vi "Example CaseStructure 2.vi"(8 "Error In":errorcluster) -> (0 "Error Out":errorcluster, 1 "signal out":waveform(dbl), 3 "appended array":waveform(dbl)[](array[waveform]))   [LabVIEW 2014]
uses:
  <vilib>/measure/NI_MABase.lvlib
panel:
  out "Boolean 3":bool
  out "Boolean 2":bool
  in  "Boolean":bool
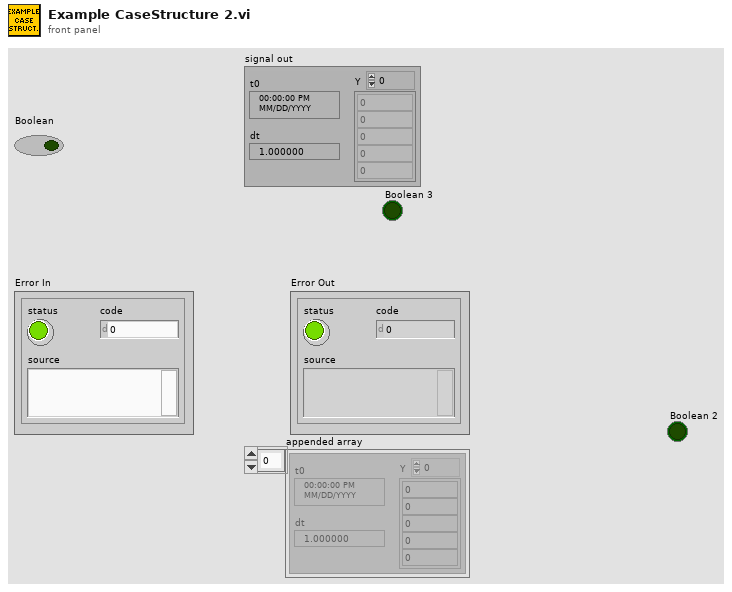
[diagram p1: front panel]
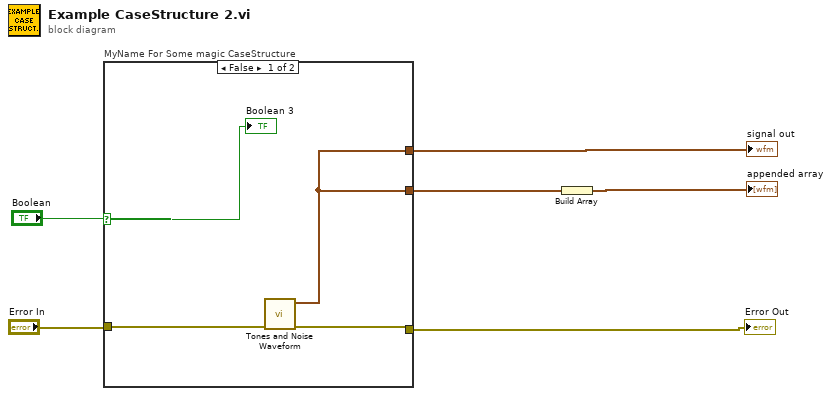
[diagram p0: block diagram]
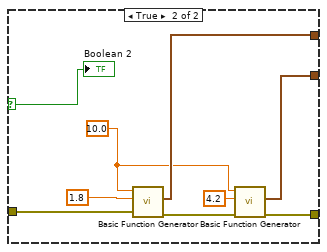
[diagram p2: hidden frame]
diagram:
  n1 = case "MyName For Some magic CaseStructure" shown="False" "Boolean" {
    selector: "Boolean" -> [w7 w11]
    tunnel: "Error In" -> [w10 w19]
    tunnel: [w9 w17] -> w1
    tunnel: [w8 w14] -> w4
    tunnel: [w8 w13] -> w3
    frame False {
      n2 = call <vilib>:"Tones and Noise Waveform.vi"("error in (no error)"=w10) -> ("error out"=w9:errorcluster, "signal out"=w8:waveform(dbl))  [unwired: 9 in]
      "Boolean 3" <- w7
    }
    frame True {
      w12 = 10.0 ("frequency")
      n3 = call <vilib>:"Basic Function Generator.vi"("error in (no error)"=w19, "amplitude"=1.8, "frequency"=w12) -> ("error out"=w18:errorcluster, "signal out"=w14:waveform(dbl))  [unwired: 6 in, 1 out]
      n4 = call <vilib>:"Basic Function Generator.vi"("error in (no error)"=w18, "amplitude"=4.2, "frequency"=w12) -> ("error out"=w17:errorcluster, "signal out"=w13:waveform(dbl))  [unwired: 6 in, 1 out]
      "Boolean 2" <- w11
    }
  }
  "Error Out" <- w1
  "signal out" <- w4
  n5 = Build Array(w3) -> (→"appended array":waveform(dbl)[])
